vi "Inverter LUT UI - Standalone.vi"() -> ()   [LabVIEW 2019]
doc: "Developed by Kevin Thompson\nkevin@thompsonengineering.net\n\nCopyright 2020\nThompson Engineering, LLC"
uses:
  DataTypes/inverter offset range--cluster.ctl
  DataTypes/inverter gain range--cluster.ctl
  <vilib>/TELLC/Dynamic CVT API/TD Dynamic CVT DVR--ref.ctl
  DataTypes/inverter info v2--cluster.ctl
  DataTypes/Inverter database record v2--cluster.ctl
  DataTypes/Inverter LUT v2--cluster.ctl
panel:
  out "last updated":string="Micro < 500W"
  in  "offset range":T1={"offset max"=3000.0, "offset min"=2000.0, "offset increment"=0.0} caption="Offset Range"
  in  "gain range":T2={"gain max"=4000.0, "gain min"=3000.0, "gain increment"=100.0} caption="Gain Range"
  in  "resistance 3 phase":dbl
  in  "resistance single phase":dbl=50.0
  in  "minimum current":dbl
  in  "power level":dbl
  in  "set flag":u16(ring) items=["False", "True"]
  in  "gain actual":dbl
  in  "offset actual":dbl
  in  "inverter Info":T3
  in  "type":string="Micro < 500W"
  in  "name":string="Inverter-01"
  in  "Inverter List":i32(listbox)
  in  "AddRec":bool
  in  "DeleteRec":bool
  out "CurrRec":i32 caption="Current\nRecord Index"
  out "Total":i32 caption="Total Inverter\nRecords"
  in  "LUT File":path
  in  "Load":bool
  in  "UpdateRec":bool
  in  "Exit":bool
  # "Inverter Record"
  # "auto filled"
  # "INVERTER  DATABASE  EDITOR"
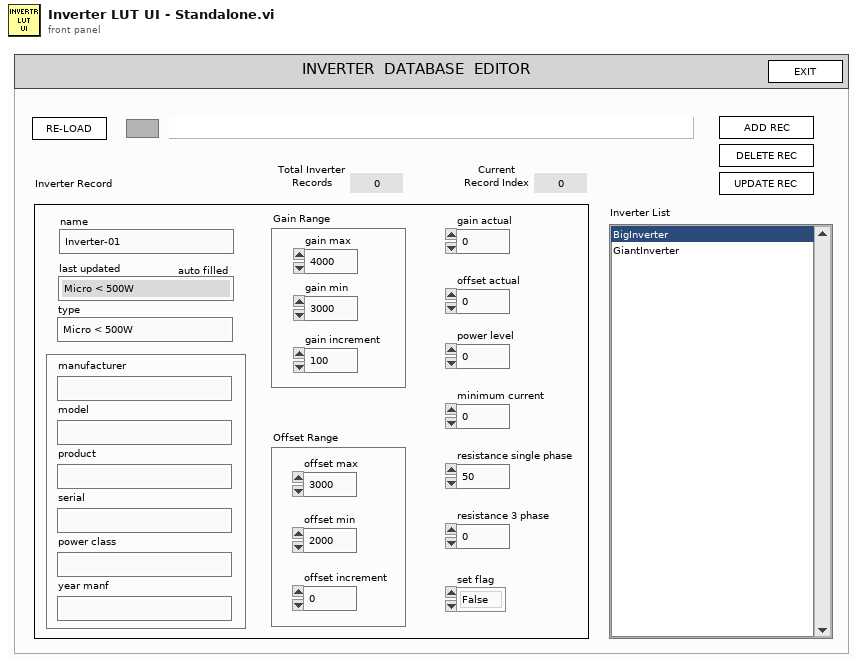
[diagram p1: front panel]
types:
  T1 = typedef "inverter offset range--cluster.ctl" = cluster{"offset max":dbl, "offset min":dbl, "offset increment":dbl}
  T2 = typedef "inverter gain range--cluster.ctl" = cluster{"gain max":dbl, "gain min":dbl, "gain increment":dbl}
  T3 = typedef "inverter info v2--cluster.ctl" = cluster{"manufacturer":string, "model":string, "product":string, "serial":string, "power class":string, "year manf":string}
  T4 = typedef "Inverter LUT v2--cluster.ctl" = cluster{"Inverter Records":T5[]}
  T5 = typedef "Inverter database record v2--cluster.ctl" = cluster{"name":string, "last updated":timestamp, "type":string, "inverter Info":T3, "gain range":T2, "offset range":T1, "gain actual":dbl, "offset actual":dbl, "power level":dbl, "minimum current":dbl, "resistance single phase":dbl, "resistance 3 phase":dbl, "set flag":u16}
  T6 = enum32{"invalid app kind", "Development System", "Run Time System", "Student Edition", "Embedded LabVIEW", "Evaluation", "Custom"}
  T7 = enum32{"Invalid", "Default", "Floating", "Floating/Auto-Hide", "Modal"}
  T8 = enum32{"Invalid", "Standard", "Closed", "Hidden", "Minimized", "Maximized"}
  T9 = typedef "TD Dynamic CVT DVR--ref.ctl" = refnum<data-value>
  T10 = cluster{"Core":cluster{"Current VI Reference":refnum<vi>, "Close Panel on Exit?":bool}, "CurrInverterRec":T5, "All Records":T5[], "InverterLUT Dict":T9}
  T11 = cluster{"Current VI Reference":refnum<vi>, "Close Panel on Exit?":bool}
  T12 = enum16{"Left Button", "Center Button", "Right Button", "Window Close"}
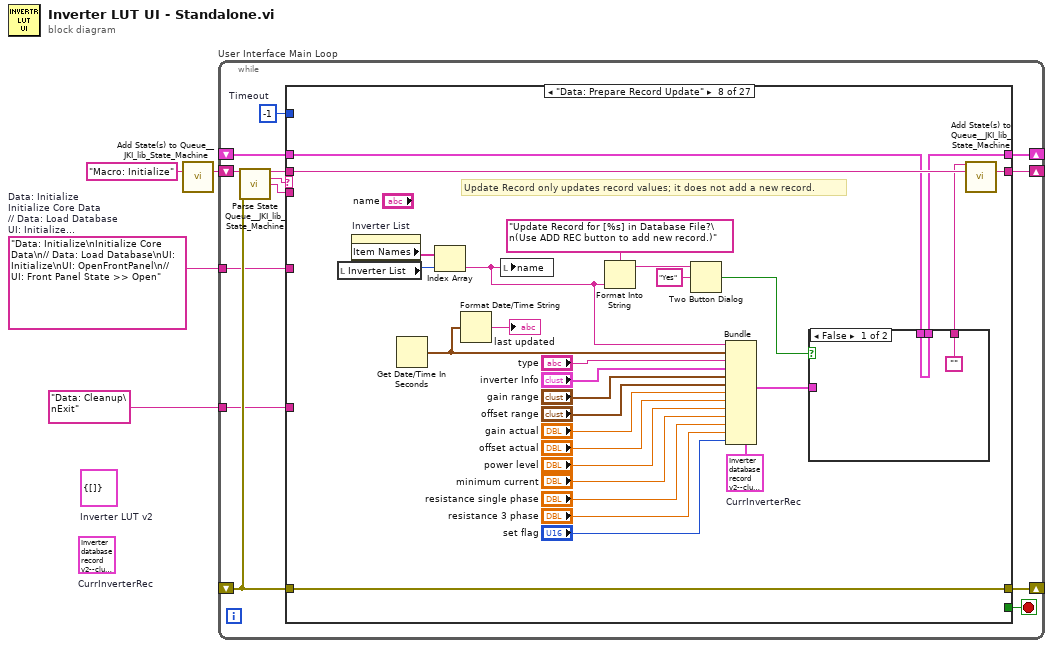
[diagram p0: block diagram]
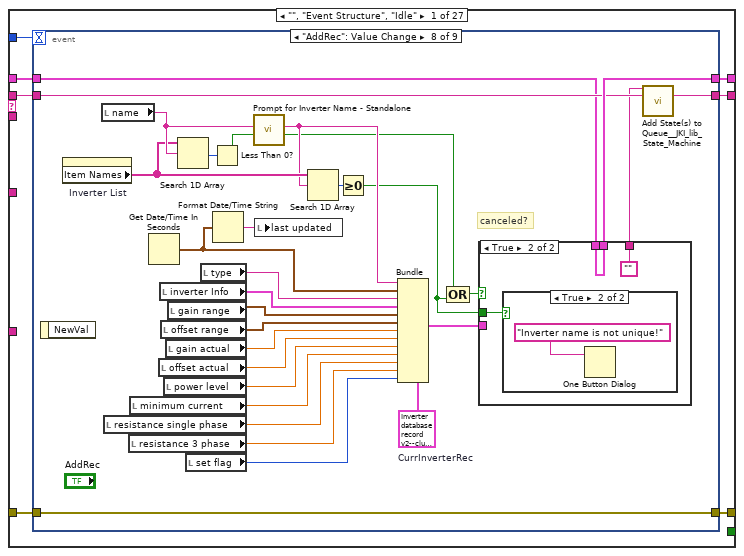
[diagram p2: hidden frame]
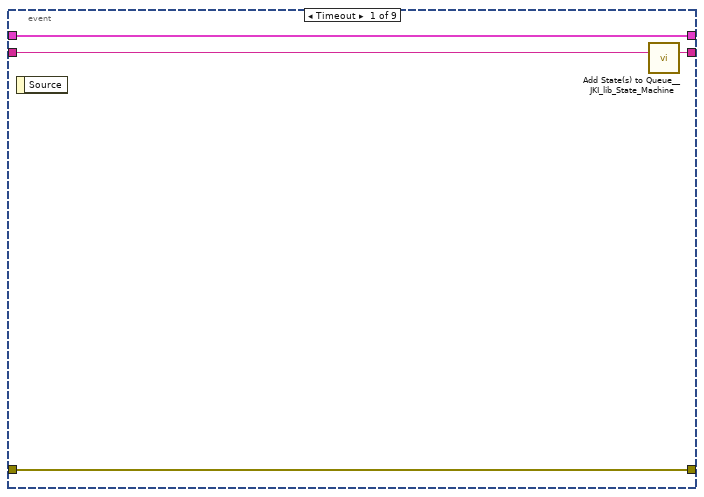
[diagram p3: hidden frame]
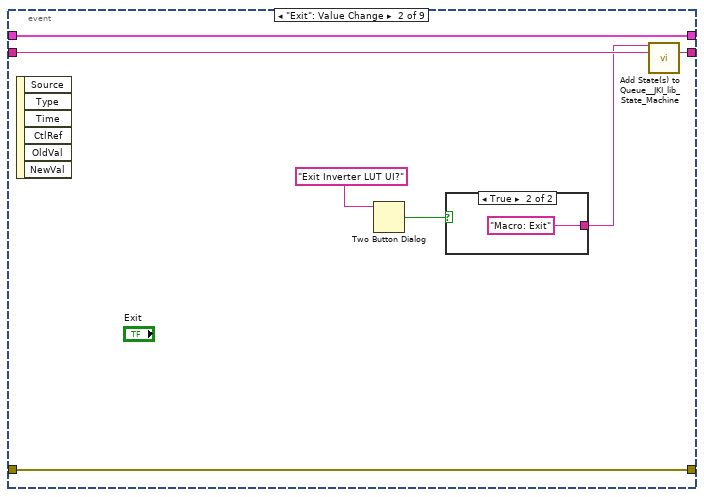
[diagram p4: hidden frame]
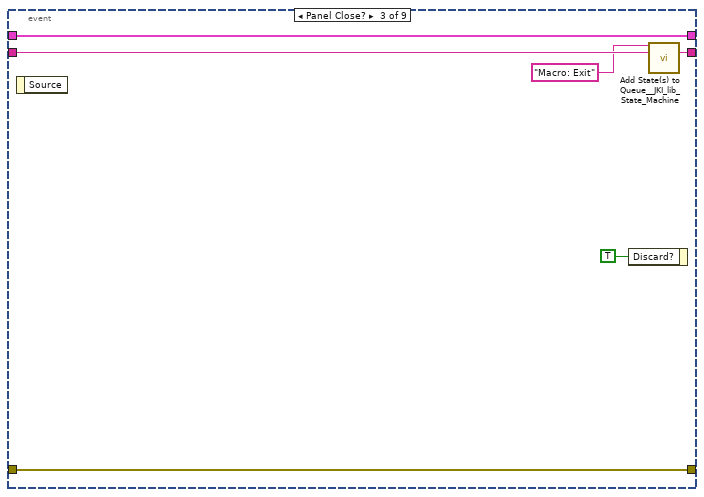
[diagram p6: hidden frame]
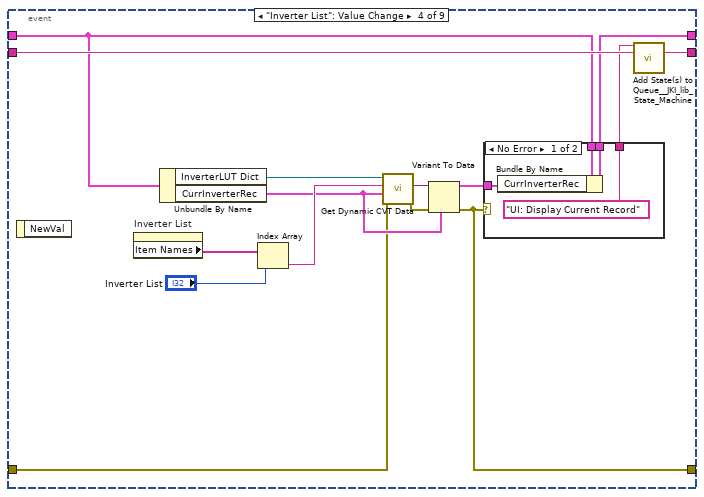
[diagram p7: hidden frame]
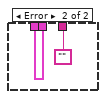
[diagram p8: hidden frame]
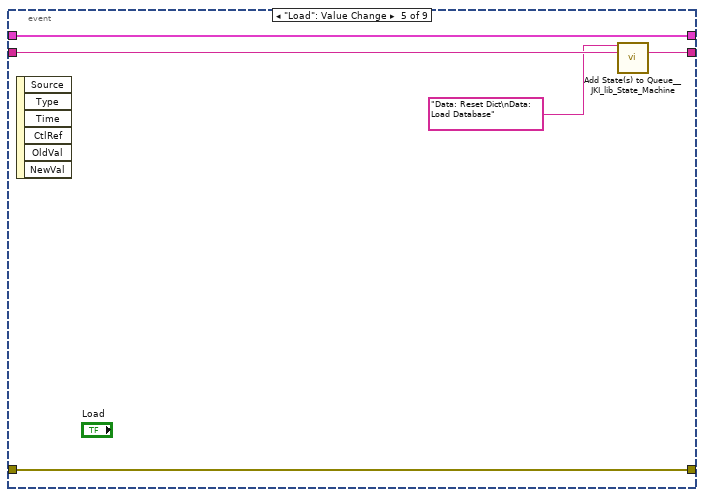
[diagram p9: hidden frame]
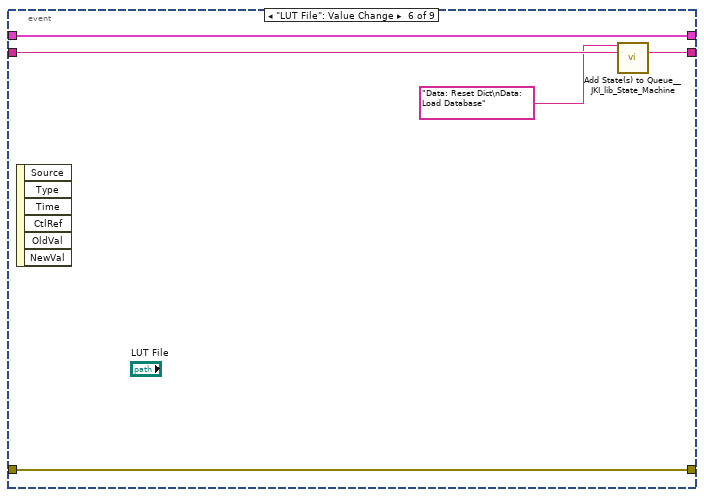
[diagram p10: hidden frame]
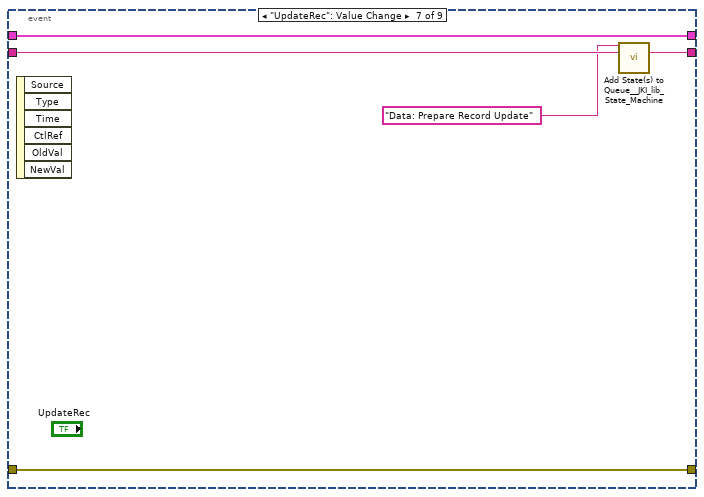
[diagram p11: hidden frame]
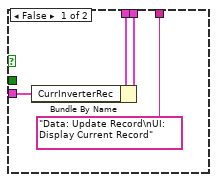
[diagram p12: hidden frame]
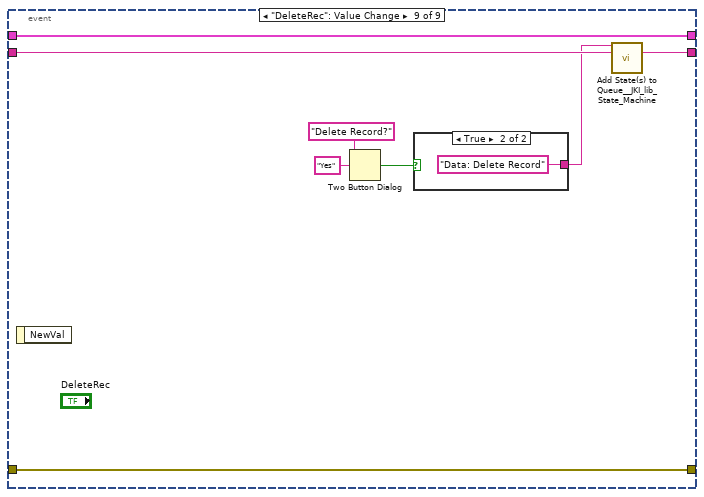
[diagram p14: hidden frame]
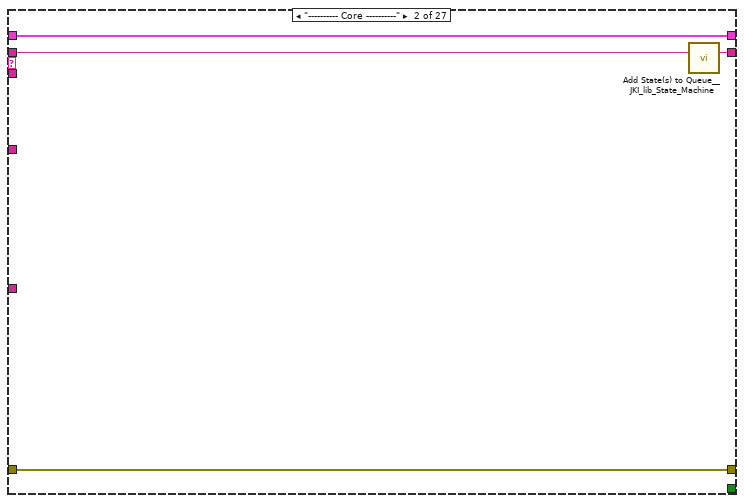
[diagram p16: hidden frame]
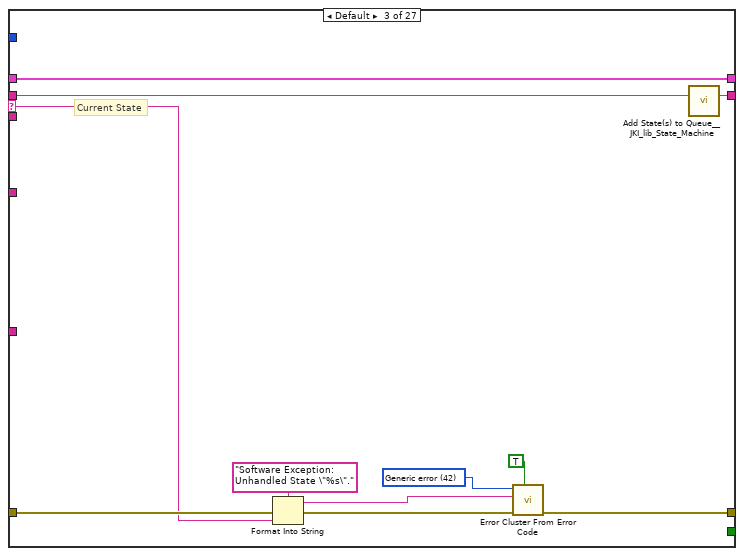
[diagram p17: hidden frame]
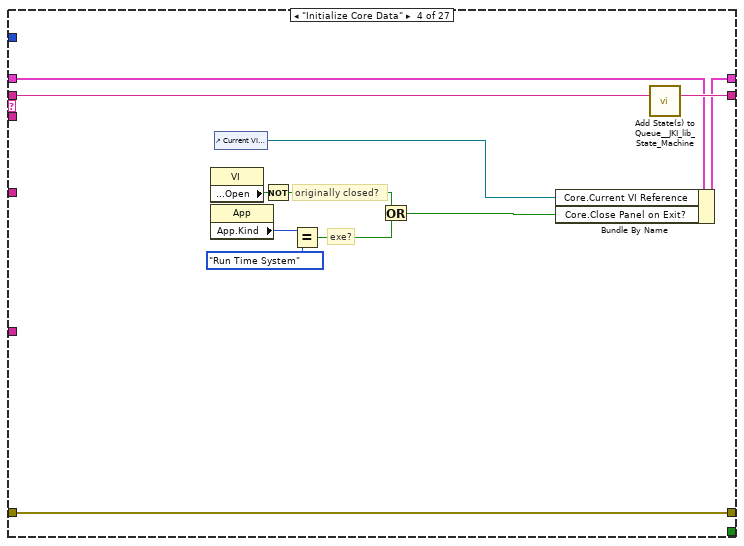
[diagram p18: hidden frame]
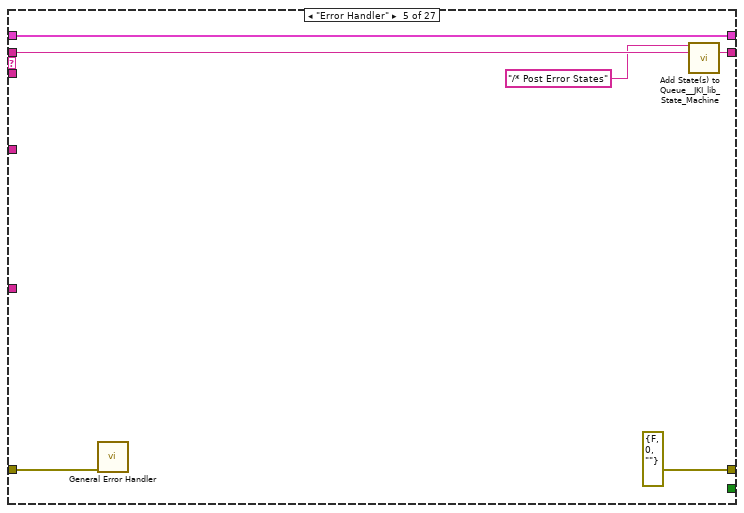
[diagram p19: hidden frame]
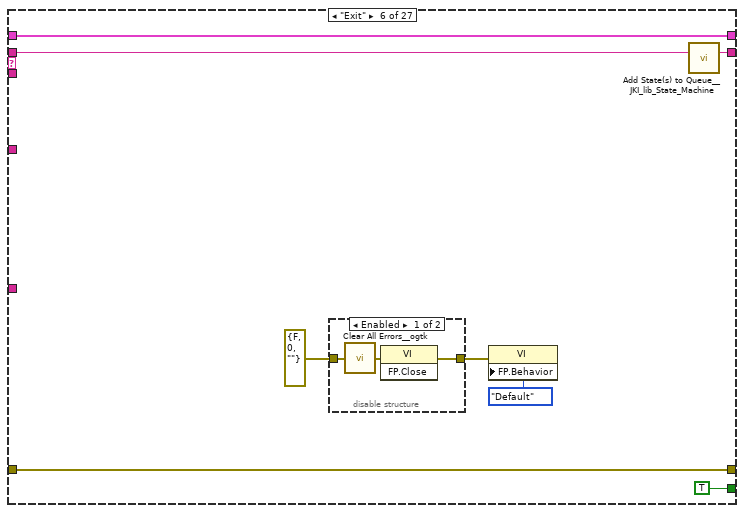
[diagram p20: hidden frame]
diagram:
  (unwired) T4 {"Inverter Records"=[]}  # Inverter LUT v2
  (unwired) T5 {"name"="", "last updated"=timestamp(0 s since 1904-01-01), "type"="", "inverter Info"={"manufacturer"="", "model"="", "product"="", "serial"="", "power class"="", "year manf"=""}, "gain range"={"gain max"=0.0, "gain min"=0.0, "gain increment"=0.0}, "offset range"={"offset max"=0.0, "offset min"=0.0, "offset increment"=0.0}, "gain actual"=0.0, "offset actual"=0.0, "power level"=0.0, "minimum current"=0.0, "resistance single phase"=0.0, "resistance 3 phase"=0.0, "set flag"=0}  # CurrInverterRec
  w2 = "Data: Initialize\nInitialize Core Data\n// Data: Load Database\nUI: Initialize\nUI: OpenFrontPanel\n// UI: Front Panel State >> Open"  # Data: Initialize Initialize Core Data // Data: Load Database UI: Initialize UI: OpenFrontPanel // UI: Front Panel State >> Open
  n1 = call <vilib>:"Add State(s) to Queue__JKI_lib_State_Machine.vi"("State(s) in (\"\")"="Macro: Initialize") -> ("States Out"=w4:string)  [unwired: 14 in]
  n2 = while "User Interface Main Loop" {
    shift-right: [w10] -> _
    shift-left: _ -> [w9]
    shift-right: [w13] -> _
    shift-left: _ -> [w7]
    shift-right: [w12] -> _
    shift-left: w4 -> [w14]
    tunnel: w2 -> [w6]
    tunnel: "Data: Cleanup\nExit" -> [w5]
    stop <- w11 stop-if-true
    w8 = -1  # Timeout
    n3 = call <vilib>:"Parse State Queue__JKI_lib_State_Machine.vi"("State Queue"=w14, "Error In (no error)"=w7) -> ("Remaining States"=w16:string, "Current State"=w17:string, "Arguments"=w15:string)  [unwired: 11 in]
    n4 = case shown="\"Data: Prepare Record Update\"" w17 {
      selector: w17 -> [_ _ w130 _ _ _ _ _ _ _ _ _ _ _ _ _ _ _ _ _ _ _ _ _ _ _ _]
      tunnel: w16 -> [w24 w129 w134 w152 w158 w166 w174 w202 w214 w234 w263 w300 w337 w346 w350 w359 w383 w405 w423 w429 w440 w466 w471 w481 w485 w489 w493]
      tunnel: w15 -> [_ _ _ _ _ _ _ _ _ _ _ _ _ _ _ _ _ _ _ w424 w434 _ _ _ _ _ _]
      tunnel: w9 -> [w22 w126 w132 w143 w155 w164 w171 w196 w212 w223 w261 w292 _ w341 w347 w356 w369 w391 w415 w427 w436 w463 w468 w478 w482 w486 w490]
      tunnel: [w21 w127 w136 w149 errorcluster {"status"=FALSE, "code"=0, "source"=""} ("error out") w163 w172 w200 w210 w218 w249 w279 w334 w342 w348 w357 w381 w403 w412 w425 w437 w464 w469 w479 w483 w487 w491] -> w13
      tunnel: w7 -> [w20 w127 w135 w149 w154 w163 w172 w200 w209 w217 w258 w293 w334 w343 w348 w357 w381 w403 w411 w426 w438 w464 w469 w479 w483 w487 w491]
      tunnel: [w23 w128 w133 w151 w157 w165 w173 w201 w213 w233 w262 w299 w336 w345 w349 w358 w382 w404 w422 w428 w439 w465 w470 w480 w484 w488 w492] -> w12
      tunnel: [_ _ _ _ _ TRUE _ _ _ _ _ _ _ _ _ _ _ _ _ _ _ _ _ _ _ _ _] -> w11
      tunnel: [w19 w126 w132 w150 w155 w164 w171 w195 w212 w224 w261 w295 w335 w341 w347 w356 w369 w391 w415 w427 w436 w463 w468 w478 w482 w486 w490] -> w10
      tunnel: w8 -> [w18 _ _ _ _ _ _ _ _ _ _ _ _ _ _ _ _ _ _ _ _ _ _ _ _ _ _]
      tunnel: w6 -> [_ _ _ _ _ _ _ _ _ _ _ _ _ _ _ _ _ _ _ _ _ _ w467 _ _ _ _]
      tunnel: w5 -> [_ _ _ _ _ _ _ _ _ _ _ _ _ _ _ _ _ _ _ _ _ _ _ w472 _ _ _]
      frame "", "Event Structure", "Idle" {
        n5 = event shown="[7] \"AddRec\": Value Change" {
          selector: _ -> [_ _ _ _ _ _ _ _ _]
          dyn-events: _ -> [_ _ _ _ _ _ _ _ _]
          timeout: w18 -> [_ _ _ _ _ _ _ _ _]
          tunnel: w24 -> [w28 w35 w42 w50 w65 w71 w76 w104 w119]
          tunnel: [w27 w34 w41 w51 w66 w72 w77 w105 w120] -> w23
          tunnel: w22 -> [w25 w32 w39 w47 w67 w69 w75 w88 w123]
          tunnel: [w26 w33 w40 w45 w68 w73 w78 w108 w124] -> w21
          tunnel: w20 -> [w26 w33 w40 w44 w68 w73 w78 w108 w124]
          tunnel: [w25 w32 w39 w48 w67 w69 w75 w107 w123] -> w19
          event Timeout {
            n6 = event-data() -> ()  [unwired: 1 in, 1 out]
            n7 = call <vilib>:"Add State(s) to Queue__JKI_lib_State_Machine.vi"("State(s) in (\"\")"=w28) -> ("States Out"=w27:string)  [unwired: 14 in]
          }
          event "Exit": Value Change {
            n8 = event-data() -> ()  [unwired: 1 in, 6 out]
            n9 = Two Button Dialog(message="Exit Inverter LUT UI?") -> (T button?=w29:bool)  [unwired: 2 in]
            n10 = case shown="True" w29 {
              tunnel: [_ "Macro: Exit"] -> w31
              frame False {
              }
              frame True {
              }
            }
            n11 = call <vilib>:"Add State(s) to Queue__JKI_lib_State_Machine.vi"("State(s) in Front (\"\")"=w31, "State(s) in (\"\")"=w35) -> ("States Out"=w34:string)  [unwired: 13 in]
          }
          event Panel Close? {
            n12 = event-data() -> ()  [unwired: 1 in, 1 out]
            n13 = event-data("Discard?"=TRUE) -> ()  [unwired: 1 in, 1 out]
            n14 = call <vilib>:"Add State(s) to Queue__JKI_lib_State_Machine.vi"("State(s) in Front (\"\")"="Macro: Exit", "State(s) in (\"\")"=w42) -> ("States Out"=w41:string)  [unwired: 13 in]
          }
          event "Inverter List": Value Change {
            n15 = event-data() -> ()  [unwired: 1 in, 1 out]
            n16 = property on="Inverter List" class="LstBox (strict)"() -> ("Item Names"=w57:string[])  [unwired: 2 in, 2 out]
            n17 = Unbundle By Name(w47) -> ("InverterLUT Dict"=w56:T9, "CurrInverterRec"=w53:T5)
            n18 = Index Array(array=w57, index="Inverter List") -> (element=w55:string)
            n19 = call <vilib>:"Get Dynamic CVT Data.vi"("error in (no error)"=w44, "default value (empty variant)"=w53, "DataName"=w55, "dCVT DVR"=w56) -> ("error out"=w54:errorcluster, "value"=w52:variant)  [unwired: 4 in, 2 out]
            n20 = Variant To Data(error in=w54, type=w53, Variant=w52) -> (data=w49:T5, error out=w45:errorcluster)
            n21 = case shown="No Error" w45 {
              tunnel: w49 -> [w61 _]
              tunnel: [w60 w63] -> w48
              tunnel: w47 -> [w59 w63]
              tunnel: ["UI: Display Current Record" ""] -> w46
              frame No Error {
                n22 = Bundle By Name(cluster=w59, "CurrInverterRec"=w61) -> (w60:T10)
              }
              frame Error {
              }
            }
            n23 = call <vilib>:"Add State(s) to Queue__JKI_lib_State_Machine.vi"("State(s) in Front (\"\")"=w46, "State(s) in (\"\")"=w50) -> ("States Out"=w51:string)  [unwired: 13 in]
          }
          event "Load": Value Change {
            n24 = event-data() -> ()  [unwired: 1 in, 6 out]
            n25 = call <vilib>:"Add State(s) to Queue__JKI_lib_State_Machine.vi"("State(s) in Front (\"\")"="Data: Reset Dict\nData: Load Database", "State(s) in (\"\")"=w65) -> ("States Out"=w66:string)  [unwired: 13 in]
          }
          event "LUT File": Value Change {
            n26 = event-data() -> ()  [unwired: 1 in, 6 out]
            n27 = call <vilib>:"Add State(s) to Queue__JKI_lib_State_Machine.vi"("State(s) in Front (\"\")"="Data: Reset Dict\nData: Load Database", "State(s) in (\"\")"=w71) -> ("States Out"=w72:string)  [unwired: 13 in]
          }
          event "UpdateRec": Value Change {
            n28 = event-data() -> ()  [unwired: 1 in, 6 out]
            n29 = call <vilib>:"Add State(s) to Queue__JKI_lib_State_Machine.vi"("State(s) in Front (\"\")"="Data: Prepare Record Update", "State(s) in (\"\")"=w76) -> ("States Out"=w77:string)  [unwired: 13 in]
          }
          event "AddRec": Value Change {
            w102 = T5 {"name"="", "last updated"=timestamp(0 s since 1904-01-01), "type"="", "inverter Info"={"manufacturer"="", "model"="", "product"="", "serial"="", "power class"="", "year manf"=""}, "gain range"={"gain max"=0.0, "gain min"=0.0, "gain increment"=0.0}, "offset range"={"offset max"=0.0, "offset min"=0.0, "offset increment"=0.0}, "gain actual"=0.0, "offset actual"=0.0, "power level"=0.0, "minimum current"=0.0, "resistance single phase"=0.0, "resistance 3 phase"=0.0, "set flag"=0}  # CurrInverterRec
            # "canceled?"
            n30 = event-data() -> ()  [unwired: 1 in, 1 out]
            n31 = property on="Inverter List" class="LstBox (strict)"() -> ("Item Names"=w84:string[])  [unwired: 2 in, 2 out]
            n32 = local read "name"() -> (w87:string)
            n33 = local read "resistance single phase"() -> (w99:dbl)
            n34 = local read "resistance 3 phase"() -> (w100:dbl)
            n35 = local read "minimum current"() -> (w98:dbl)
            n36 = Get Date/Time In Seconds() -> (seconds since 1Jan1904=w90:timestamp)
            n37 = local read "offset actual"() -> (w96:dbl)
            n38 = local read "inverter Info"() -> (w92:T3)
            n39 = local read "offset range"() -> (w94:T1)
            n40 = local read "power level"() -> (w97:dbl)
            n41 = local read "gain actual"() -> (w95:dbl)
            n42 = local read "gain range"() -> (w93:T2)
            n43 = Search 1D Array(1D array=w84, element=w87) -> (index of element=w86:i32)  [unwired: 1 in]
            n44 = local read "set flag"() -> (w101:u16)
            n45 = local read "type"() -> (w91:string)
            n46 = Less Than 0?(x=w86) -> (x < 0?=w85:bool)
            n47 = Format Date/Time String(seconds (now)=w90) -> (date/time string=w89:string)  [unwired: 2 in]
            n48 = call "Prompt for Inverter Name - Standalone.vi"("bypass (F)"=w85, "Name"=w87) -> ("canceled"=w80:bool, "name out"=w83:string)  [unwired: 7 in, 1 out]
            n49 = local write "last updated"(w89) -> ()
            n50 = Search 1D Array(1D array=w84, element=w83) -> (index of element=w82:i32)  [unwired: 1 in]
            n51 = Greater Or Equal To 0?(x=w82) -> (x >= 0?=w79:bool)
            n52 = Bundle(cluster=w102, "name"=w83, "last updated"=w90, "type"=w91, "inverter Info"=w92, "gain range"=w93, "offset range"=w94, "gain actual"=w95, "offset actual"=w96, "power level"=w97, "minimum current"=w98, "resistance single phase"=w99, "resistance 3 phase"=w100, "set flag"=w101) -> (w106:T5)
            n53 = Compound Arithmetic op=OR(w80, w79) -> (w81:bool)
            n54 = case shown="True" w81 {
              tunnel: [w112 w115] -> w107
              tunnel: w88 -> [w111 w115]
              tunnel: w106 -> [w110 _]
              tunnel: ["Data: Update Record\nUI: Display Current Record" ""] -> w103
              tunnel: w79 -> [_ w113]
              frame False {
                n55 = Bundle By Name(cluster=w111, "CurrInverterRec"=w110) -> (w112:T10)
              }
              frame True {
                n56 = case shown="True" w113 {
                  frame False {
                  }
                  frame True {
                    n57 = One Button Dialog(message="Inverter name is not unique!") -> ()  [unwired: 1 in, 1 out]
                  }
                }
              }
            }
            n58 = call <vilib>:"Add State(s) to Queue__JKI_lib_State_Machine.vi"("State(s) in Front (\"\")"=w103, "State(s) in (\"\")"=w104) -> ("States Out"=w105:string)  [unwired: 13 in]
          }
          event "DeleteRec": Value Change {
            n59 = event-data() -> ()  [unwired: 1 in, 1 out]
            n60 = Two Button Dialog(message="Delete Record?", 2:"Yes" ("T button name (\"OK\")")) -> (T button?=w117:bool)  [unwired: 1 in]
            n61 = case shown="True" w117 {
              tunnel: [_ "Data: Delete Record"] -> w118
              frame False {
              }
              frame True {
              }
            }
            n62 = call <vilib>:"Add State(s) to Queue__JKI_lib_State_Machine.vi"("State(s) in Front (\"\")"=w118, "State(s) in (\"\")"=w119) -> ("States Out"=w120:string)  [unwired: 13 in]
          }
        }
      }
      frame "---------- Core ----------" {
        n63 = call <vilib>:"Add State(s) to Queue__JKI_lib_State_Machine.vi"("State(s) in (\"\")"=w129) -> ("States Out"=w128:string)  [unwired: 14 in]
      }
      frame Default {
        w139 = 42 items=["No error", "Argument error", "Memory is full", "Out of zone", "End of file", "File already open", "Generic file I/O error", "File not found", "File permission error", "Disk is full", "Duplicate path", "Too many files open", "System feature not enabled", "Resource file not found", "Cannot add resource", "Resource not found", "Image not found", "Image memory error", "Pen does not exist", "Config type invalid", "Config token not found", "Config parse error", "Config memory error", "Bad external code format", "Bad external code offset", "External code not present", "Null window", "Destroy window error", "Null menu", "Print aborted", "Bad print record", "Print driver error", "Windows error during printing", "Memory error during printing", "Print dialog error", "Generic print error", "Invalid device refnum", "Device not found", "Device parameter error", "Device unit error", "Cannot open device", "Device call aborted", "Generic error", "Cancelled by user", "Object ID too low", "Object ID too high", "Object not in heap", "Unknown heap", "Unknown object (invalid DefProc)", "Unknown object (DefProc not in table)", "Message out of range", "Invalid (null) method", "Unknown message", "Manager call not supported", "Bad address", "Network operation in progress", "Network operation timed out", "Connection is busy", "Network attribute not supported", "Network error", "Address in use", "System out of memory", "Connection aborted", "Connection refused", "Not connected", "Already connected", "Connection closed", "Initialization error (interapplication manager)", "Bad occurrence", "Wait on unbound occurrence handler", "Occurrence queue overflow", "Datalog type conflict", "Unused", "Unrecognized type (interapplication manager)", "Memory corrupt", "Failed to make temporary DLL", "Old CIN version", "Drag socket not found", "Failed to load drop-object", "Failed to register OLE object", "Failed to release OLE object", "Format specifier type mismatch", "Unknown format specifier", "Too few format specifiers", "Too many format specifiers", "Scan failed", "Newer CIN version", "Error converting to variant", "Runtime menu error", "Password tampered", "Variant attribute not found", "Incompatible variant data type", "Event data is not available", "Event Store is not present", "Occurrence is not found", "Event Queue is not created", "Event info is not available", "Refnum passed is NULL", "Error retrieving Class GUID", "Error retrieving CoClass GUID", "Error retrieving TypeLib GUID.", "Bad built application magic bytes.", "Specific driver is different from the specific driver associated with the Logical Name.", "There is no session opened to the class driver.", "Max Error", "MAX - Error with config objects", "MAX - Error loading configuration", "MAX - Group not supported"]
        # "Current State"
        n64 = Format Into String(format string="Software Exception: Unhandled State \"%s\"." ("message"), error in=w135, w130) -> (resulting string=w138:string, error out=w137:errorcluster)  [unwired: 1 in]
        n65 = call <vilib>:"Error Cluster From Error Code.vi"("show call chain? (False)"=TRUE, "error in (no error)"=w137, "error message (\"\")"=w138, "error code (0)"=w139) -> ("error out"=w136:errorcluster)  [unwired: 5 in]
        n66 = call <vilib>:"Add State(s) to Queue__JKI_lib_State_Machine.vi"("State(s) in (\"\")"=w134) -> ("States Out"=w133:string)  [unwired: 14 in]
      }
      frame "Initialize Core Data" {
        # "originally closed?"
        # "exe?"
        n67 = property class="VI"() -> ("Front Panel.Open"=w148:bool)  [unwired: 2 in, 2 out]
        n68 = property class="App"() -> ("App.Kind"=w147:T6)  [unwired: 2 in, 2 out]
        n69 = control-ref of="Current VI Reference"() -> (w141:refnum<vi>)
        n70 = Not(x=w148) -> (.not. x?=w145:bool)
        n71 = Equal?(x=w147, y=T6."Run Time System" ("Application:Kind")) -> (x = y?=w144:bool)
        n72 = Or(x=w145, y=w144) -> (x .or. y?=w142:bool)
        n73 = Bundle By Name(cluster=w143, "Core.Current VI Reference"=w141, "Core.Close Panel on Exit?"=w142) -> (w150:T10)
        n74 = call <vilib>:"Add State(s) to Queue__JKI_lib_State_Machine.vi"("State(s) in (\"\")"=w152) -> ("States Out"=w151:string)  [unwired: 14 in]
      }
      frame "Error Handler" {
        n75 = call <vilib>:"General Error Handler.vi"("error in (no error)"=w154) -> ()  [unwired: 10 in, 5 out]
        n76 = call <vilib>:"Add State(s) to Queue__JKI_lib_State_Machine.vi"("State(s) in Front (\"\")"="/* Post Error States", "State(s) in (\"\")"=w158) -> ("States Out"=w157:string)  [unwired: 13 in]
      }
      frame "Exit" {
        n77 = disable-structure shown="Enabled" {
          disable-tunnel: [w169 w170] -> w161
          disable-tunnel: errorcluster {"status"=FALSE, "code"=0, "source"=""} ("Error In") -> [w167 w170]
          frame Enabled {
            n78 = call <userlib>:"Clear All Errors__ogtk.vi"("Error In"=w167) -> ("Error Out"=w168:errorcluster)  [unwired: 3 in]
            n79 = invoke class="VI" method="FP.Close"(error in=w168) -> (error out=w169:errorcluster)  [unwired: 2 in, 2 out]
          }
          frame Disabled {
          }
        }
        n80 = property class="VI"(error in=w161, "FP.Behavior"=T7."Default" ("Front Panel Window:Behavior")) -> ()  [unwired: 1 in, 2 out]
        n81 = call <vilib>:"Add State(s) to Queue__JKI_lib_State_Machine.vi"("State(s) in (\"\")"=w166) -> ("States Out"=w165:string)  [unwired: 14 in]
      }
      frame "---------- Data ----------" {
        n82 = call <vilib>:"Add State(s) to Queue__JKI_lib_State_Machine.vi"("State(s) in (\"\")"=w174) -> ("States Out"=w173:string)  [unwired: 14 in]
      }
      frame "Data: Prepare Record Update" {
        w189 = T5 {"name"="", "last updated"=timestamp(0 s since 1904-01-01), "type"="", "inverter Info"={"manufacturer"="", "model"="", "product"="", "serial"="", "power class"="", "year manf"=""}, "gain range"={"gain max"=0.0, "gain min"=0.0, "gain increment"=0.0}, "offset range"={"offset max"=0.0, "offset min"=0.0, "offset increment"=0.0}, "gain actual"=0.0, "offset actual"=0.0, "power level"=0.0, "minimum current"=0.0, "resistance single phase"=0.0, "resistance 3 phase"=0.0, "set flag"=0}  # CurrInverterRec
        # "Update Record only updates record values; it does not add a new record."
        n83 = local read "Inverter List"() -> (w193:i32)
        n84 = property on="Inverter List" class="LstBox (strict)"() -> ("Item Names"=w192:string[])  [unwired: 2 in, 2 out]
        n85 = Get Date/Time In Seconds() -> (seconds since 1Jan1904=w175:timestamp)
        n86 = Index Array(array=w192, index=w193) -> (element=w177:string)
        n87 = Format Date/Time String(seconds (now)=w175) -> (date/time string=→"last updated":string)  [unwired: 2 in]
        n88 = local write "name"(w177) -> ()
        n89 = Format Into String(format string="Update Record for [%s] in Database File?\n(Use ADD REC button to add new record.)" ("message"), w177) -> (resulting string=w190:string)  [unwired: 2 in, 1 out]
        n90 = Two Button Dialog(message=w190, 2:"Yes" ("T button name (\"OK\")")) -> (T button?=w198:bool)  [unwired: 1 in]
        n91 = Bundle(cluster=w189, "name"=w177, "last updated"=w175, "type"="type", "inverter Info"="inverter Info", "gain range"="gain range", "offset range"="offset range", "gain actual"="gain actual", "offset actual"="offset actual", "power level"="power level", "minimum current"="minimum current", "resistance single phase"="resistance single phase", "resistance 3 phase"="resistance 3 phase", "set flag"="set flag") -> (w199:T5)
        n92 = case shown="False" w198 {
          tunnel: [w204 w208] -> w195
          tunnel: w196 -> [w204 w207]
          tunnel: w199 -> [_ w206]
          tunnel: ["" "Data: Update Record"] -> w194
          frame False {
          }
          frame True {
            n93 = Bundle By Name(cluster=w207, "CurrInverterRec"=w206) -> (w208:T10)
          }
        }
        n94 = call <vilib>:"Add State(s) to Queue__JKI_lib_State_Machine.vi"("State(s) in Front (\"\")"=w194, "State(s) in (\"\")"=w202) -> ("States Out"=w201:string)  [unwired: 13 in]
      }
      frame "Data: Reset Dict" {
        n95 = Unbundle By Name(w212) -> ("InverterLUT Dict"=w211:T9)
        n96 = call <vilib>:"Delete ALL Dynamic CVT Data.vi"("error in (no error)"=w209, "dCVT DVR"=w211) -> ("error out"=w210:errorcluster)  [unwired: 8 in, 1 out]
        n97 = call <vilib>:"Add State(s) to Queue__JKI_lib_State_Machine.vi"("State(s) in (\"\")"=w214) -> ("States Out"=w213:string)  [unwired: 14 in]
      }
      frame "Data: Delete Record" {
        w215 = T5 {"name"="", "last updated"=timestamp(0 s since 1904-01-01), "type"="", "inverter Info"={"manufacturer"="", "model"="", "product"="", "serial"="", "power class"="", "year manf"=""}, "gain range"={"gain max"=0.0, "gain min"=0.0, "gain increment"=0.0}, "offset range"={"offset max"=0.0, "offset min"=0.0, "offset increment"=0.0}, "gain actual"=0.0, "offset actual"=0.0, "power level"=0.0, "minimum current"=0.0, "resistance single phase"=0.0, "resistance 3 phase"=0.0, "set flag"=0}  # CurrInverterRec
        n98 = Unbundle By Name(w223) -> ("InverterLUT Dict"=w232:T9, "CurrInverterRec"=w230:T5)
        n99 = Unbundle By Name(w230) -> ("name"=w231:string)
        n100 = call <vilib>:"Delete Dynamic CVT Data.vi"("error in (no error)"=w217, "DataName"=w231, "dCVT DVR"=w232) -> ("error out"=w228:errorcluster, "CVT DVR out"=w229:T9)  [unwired: 6 in, 1 out]
        n101 = call <vilib>:"Get ALL Dynamic CVT Data.vi"("error in (no error)"=w228, "dCVT DVR"=w229) -> ("error out"=w220:errorcluster, "NameArray"=w225:string[], "ValueArray"=w227:variant[])  [unwired: 6 in, 1 out]
        n102 = Index Array(array=w227) -> (element=w226:variant)  [unwired: 1 in]
        n103 = property on="Inverter List" class="LstBox (strict)"(error in=w220, "Item Names"=w225) -> (error out=w221:errorcluster)  [unwired: 1 in, 1 out]
        n104 = Variant To Data(error in=w220, type=w215, Variant=w226) -> (data=w222:T5, error out=w219:errorcluster)
        n105 = Bundle By Name(cluster=w223, "CurrInverterRec"=w222) -> (w224:T10)
        n106 = flat-sequence {
          tunnel: w221 -> [w237]
          tunnel: w219 -> [w236]
          tunnel: [w235] -> w218
          frame #0 {
            n107 = Merge Errors(w236, w237) -> (w235:errorcluster)
            n108 = local write "Inverter List"(0 ("Inverter List")) -> ()
          }
        }
        n109 = call <vilib>:"Add State(s) to Queue__JKI_lib_State_Machine.vi"("State(s) in Front (\"\")"="Data: Update Record\nUI: Display Current Record", "State(s) in (\"\")"=w234) -> ("States Out"=w233:string)  [unwired: 13 in]
      }
      frame "Data: Update Record" {
        w239 = T4 {"Inverter Records"=[]}  # Inverter LUT v2
        n110 = Unbundle By Name(w261) -> ("InverterLUT Dict"=w260:T9, "CurrInverterRec"=w259:T5)
        n111 = Unbundle By Name(w259) -> ("name"=w247:string)
        n112 = call <vilib>:"Set Dynamic CVT Data.vi"("error in (no error)"=w258, "value"=w259, "DataName"=w247, "dCVT DVR"=w260) -> ("error out"=w256:errorcluster, "dCVT DVR out"=w257:T9)  [unwired: 5 in, 1 out]
        n113 = call <userlib>:"Clear All Errors__ogtk.vi"("Error In"=w256) -> ("Error Out"=w241:errorcluster)  [unwired: 3 in]
        n114 = call <vilib>:"Get ALL Dynamic CVT Data.vi"("error in (no error)"=w241, "dCVT DVR"=w257) -> ("error out"=w250:errorcluster, "NameArray"=w248:string[], "ValueArray"=w255:variant[])  [unwired: 6 in, 1 out]
        n115 = call <userlib>:"Clear All Errors__ogtk.vi"("Error In"=w250) -> ("Error Out"=w240:errorcluster)  [unwired: 3 in]
        n116 = for {
          tunnel: w255 -> [w272] mode=indexing
          tunnel: [w271] -> w254 mode=indexing
          n117 = Variant To Data(type=T5 {"name"="", "last updated"=timestamp(0 s since 1904-01-01), "type"="", "inverter Info"={"manufacturer"="", "model"="", "product"="", "serial"="", "power class"="", "year manf"=""}, "gain range"={"gain max"=0.0, "gain min"=0.0, "gain increment"=0.0}, "offset range"={"offset max"=0.0, "offset min"=0.0, "offset increment"=0.0}, "gain actual"=0.0, "offset actual"=0.0, "power level"=0.0, "minimum current"=0.0, "resistance single phase"=0.0, "resistance 3 phase"=0.0, "set flag"=0} ("CurrInverterRec"), Variant=w272) -> (data=w271:T5)  [unwired: 1 in, 1 out]
        }
        n118 = Array Size(array=w248) -> (size(s)=→"Total":i32)
        n119 = Search 1D Array(1D array=w248, element=w247) -> (index of element=w246:i32)  [unwired: 1 in]
        n120 = property on="Inverter List" class="LstBox (strict)"("Item Names"=w248) -> ()  [unwired: 2 in, 2 out]
        n121 = local write "Inverter List"(w246) -> ()
        n122 = Variant To Data(type=T5[] [] ("Inverter Records"), Variant=w254) -> (data=w252:T5[])  [unwired: 1 in, 1 out]
        n123 = Bundle(cluster=w239, "Inverter Records"=w252) -> (w251:T4)
        n124 = local read "LUT File"() -> (w243:path)
        n125 = Empty String/Path?(string/path=w243) -> (empty?=w242:bool)
        n126 = Increment(x=w246) -> (x+1=→"CurrRec":i32)
        n127 = case shown="False" w242 {
          tunnel: w251 -> [w268 _]
          tunnel: w240 -> [w266 w269]
          tunnel: [w265 w269] -> w249
          tunnel: w243 -> [w264 _]
          frame False {
            n128 = call <vilib>:"Easy Write XML File__JKI EasyXML.vi"("error in (no error)"=w266, "Overwrite File? (false)"=TRUE, "LabVIEW Data"=w268, "XML File Path"=w264) -> ("error out"=w265:errorcluster)  [unwired: 6 in, 1 out]
          }
          frame True {
          }
        }
        n129 = call <vilib>:"Add State(s) to Queue__JKI_lib_State_Machine.vi"("State(s) in (\"\")"=w263) -> ("States Out"=w262:string)  [unwired: 14 in]
      }
      frame "Data: Load Database" {
        w284 = T4 {"Inverter Records"=[]}  # Inverter LUT v2
        # "Size difference indicates database file\nhad some duplicate inverter names;\nwhich is not allowed."
        n130 = local read "LUT File"() -> (w285:path)
        n131 = Unbundle By Name(w292) -> ("InverterLUT Dict"=w291:T9)
        n132 = call <vilib>:"Easy Read XML File__JKI EasyXML.vi"("error in (no error)"=w293, "LabVIEW Data (Type)"=w284, "XML File Path"=w285) -> ("error out"=w298:errorcluster, "LabVIEW Data"=w297:variant)  [unwired: 6 in, 1 out]
        n133 = Variant To Data(error in=w298, type=w284, Variant=w297) -> (data=w296:T4, error out=w290:errorcluster)
        n134 = Unbundle(w296) -> ("Inverter Records"=w276:T5[])
        n135 = Array Size(array=w276) -> (size(s)=w275:i32)
        n136 = for {
          tunnel: w276 -> [w316] mode=indexing
          shift-right: [w317] -> w282
          shift-left: w290 -> [w318]
          shift-right: [w319] -> w283
          shift-left: w291 -> [w320]
          n137 = Unbundle By Name(w316) -> ("name"=w315:string)
          n138 = call <vilib>:"Set Dynamic CVT Data.vi"("error in (no error)"=w318, "value"=w316, "DataName"=w315, "dCVT DVR"=w320) -> ("error out"=w317:errorcluster, "dCVT DVR out"=w319:T9)  [unwired: 5 in, 1 out]
        }
        n139 = call <vilib>:"Get ALL Dynamic CVT Data.vi"("error in (no error)"=w282, "dCVT DVR"=w283) -> ("error out"=w280:errorcluster, "NameArray"=w278:string[], "ValueArray"=w281:variant[])  [unwired: 6 in, 1 out]
        n140 = for {
          tunnel: w281 -> [w305] mode=indexing
          tunnel: [w303] -> w277 mode=indexing
          shift-right: [w301] -> w279
          shift-left: w280 -> [w302]
          w304 = T5 {"name"="", "last updated"=timestamp(0 s since 1904-01-01), "type"="", "inverter Info"={"manufacturer"="", "model"="", "product"="", "serial"="", "power class"="", "year manf"=""}, "gain range"={"gain max"=0.0, "gain min"=0.0, "gain increment"=0.0}, "offset range"={"offset max"=0.0, "offset min"=0.0, "offset increment"=0.0}, "gain actual"=0.0, "offset actual"=0.0, "power level"=0.0, "minimum current"=0.0, "resistance single phase"=0.0, "resistance 3 phase"=0.0, "set flag"=0}  # CurrInverterRec
          n141 = Variant To Data(error in=w302, type=w304, Variant=w305) -> (data=w303:T5, error out=w301:errorcluster)
        }
        n142 = Array Size(array=w277) -> (size(s)=w274:i32)
        n143 = local write "Total"(w274) -> ()
        n144 = Not Equal?(x=w275, y=w274) -> (x != y?=w273:bool)
        n145 = Greater Than 0?(x=w274) -> (x > 0?=w289:bool)
        n146 = case shown="True" w289 {
          tunnel: ["" w312] -> w287
          tunnel: [0 ("CurrRec") 1 ("CurrRec")] -> w288
          tunnel: [-1 ("Inverter List") 0 ("Inverter List")] -> w286
          tunnel: w273 -> [_ w309]
          frame False {
          }
          frame True {
            n147 = case shown="True" w309 {
              tunnel: ["UI: Display Current Record" "UI: Warn Dup Records Eliminated"] -> w312
              frame False {
              }
              frame True {
              }
            }
          }
        }
        n148 = Index Array(array=w277) -> (element=w294:T5)  [unwired: 1 in]
        n149 = property on="Inverter List" class="LstBox (strict)"("Item Names"=w278) -> ()  [unwired: 2 in, 2 out]
        n150 = Bundle By Name(cluster=w292, "All Records"=w277, "CurrInverterRec"=w294) -> (w295:T10)
        n151 = local write "CurrRec"(w288) -> ()
        n152 = local write "Inverter List"(w286) -> ()
        n153 = call <vilib>:"Add State(s) to Queue__JKI_lib_State_Machine.vi"("State(s) in Front (\"\")"=w287, "State(s) in (\"\")"=w300) -> ("States Out"=w299:string)  [unwired: 13 in]
      }
      frame "Data: Initialize" {
        w323 = T5 {"name"="", "last updated"=timestamp(0 s since 1904-01-01), "type"="", "inverter Info"={"manufacturer"="", "model"="", "product"="", "serial"="", "power class"="", "year manf"=""}, "gain range"={"gain max"=0.0, "gain min"=0.0, "gain increment"=0.0}, "offset range"={"offset max"=0.0, "offset min"=0.0, "offset increment"=0.0}, "gain actual"=0.0, "offset actual"=0.0, "power level"=0.0, "minimum current"=0.0, "resistance single phase"=0.0, "resistance 3 phase"=0.0, "set flag"=0}  # CurrInverterRec
        w325 = string[] []  # InverterNames[]
        w328 = T5[] []  # All Records
        w329 = T9 refnum  # InverterLUT Dict
        w333 = T11 {"Current VI Reference"=refnum, "Close Panel on Exit?"=FALSE}  # Core
        n154 = Get Date/Time In Seconds() -> (seconds since 1Jan1904=w321:timestamp)
        n155 = local write "LUT File"(path "" ("LUT File")) -> ()
        n156 = Bundle By Name(cluster=w323, "last updated"=w321) -> (w322:T5)
        n157 = Initialize Array(w322, 0 ("dimension size")) -> (w327:T5[])
        n158 = Variant To Data(type=w328, Variant=w327) -> (data=w332:T5[])  [unwired: 1 in, 1 out]
        n159 = call <vilib>:"Create Dynamic CVT Reference.vi"() -> ("dCVT DVR out"=w331:T9)  [unwired: 10 in, 1 out]
        n160 = property on="Inverter List" class="LstBox (strict)"("Item Names"=w325) -> ()  [unwired: 2 in, 2 out]
        n161 = Variant To Data(type=w329, Variant=w331) -> (data=w330:T9)  [unwired: 1 in, 1 out]
        n162 = Bundle("Core"=w333, "CurrInverterRec"=w322, "All Records"=w332, "InverterLUT Dict"=w330) -> (w335:T10)  [unwired: 1 in]
        n163 = call <vilib>:"Add State(s) to Queue__JKI_lib_State_Machine.vi"("State(s) in (\"\")"=w337) -> ("States Out"=w336:string)  [unwired: 14 in]
      }
      frame "Data: Cleanup" {
        n164 = Unbundle By Name(w341) -> ("InverterLUT Dict"=w340:T9, "Core.Current VI Reference"=w344:refnum<vi>)
        n165 = Close Reference(reference=w344, error in (no error)=w343) -> (error out=w342:errorcluster)
        n166 = call <vilib>:"Delete ALL Dynamic CVT Data.vi"("dCVT DVR"=w340) -> ("error out"=w338:errorcluster, "dCVT DVR out"=w339:T9)  [unwired: 9 in]
        n167 = call <vilib>:"Destroy Dynamic CVT Reference.vi"("error in (no error)"=w338, "dCVT DVR"=w339) -> ()  [unwired: 8 in, 2 out]
        n168 = call <vilib>:"Add State(s) to Queue__JKI_lib_State_Machine.vi"("State(s) in (\"\")"=w346) -> ("States Out"=w345:string)  [unwired: 14 in]
      }
      frame "---------- UI ----------" {
        n169 = call <vilib>:"Add State(s) to Queue__JKI_lib_State_Machine.vi"("State(s) in (\"\")"=w350) -> ("States Out"=w349:string)  [unwired: 14 in]
      }
      frame "UI: Warn Dup Records Eliminated" {
        n170 = call <vilib>:"Three Button Dialog.vi"("Window Title (\"\")"="WARNING" ("Window Title (\"\")"), "Center Button Text (\"No\")"="", "message"="Warning: Some records had duplicate Inverter Names.\nInverter Names in the database must be unique.\n\nProceed to update database file with duplicate names removed?\n\nNote: \n<Cancel> terminates editor, and does not modify the database file.\n<Yes> Updates the database file with duplicate Inverter Name records eliminated.") -> ("Which Button?"=w352:T12)  [unwired: 8 in]
        n171 = case shown="\"Left Button\"" w352 {
          tunnel: ["Macro: Exit" "Data: Update Record\nUI: Display Current Record"] -> w351
          frame Default {
          }
          frame "Left Button" {
          }
        }
        n172 = call <vilib>:"Add State(s) to Queue__JKI_lib_State_Machine.vi"("State(s) in Front (\"\")"=w351, "State(s) in (\"\")"=w359) -> ("States Out"=w358:string)  [unwired: 13 in]
      }
      frame "UI: Display Current Record" {
        n173 = Unbundle By Name(w369) -> ("CurrInverterRec"=w368:T5)
        n174 = Unbundle By Name(w368) -> ("name"=w367:string, "last updated"=w362:timestamp, "type"=w380:string, "inverter Info"=w379:T3, "gain range"=w378:T2, "offset range"=w377:T1, "gain actual"=w376:dbl, "offset actual"=w375:dbl, "power level"=w373:dbl, "minimum current"=w374:dbl, "resistance single phase"=w372:dbl, "resistance 3 phase"=w371:dbl, "set flag"=w370:u16)
        n175 = property on="Inverter List" class="LstBox (strict)"() -> ("Item Names"=w366:string[])  [unwired: 2 in, 2 out]
        n176 = local write "inverter Info"(w379) -> ()
        n177 = local write "offset range"(w377) -> ()
        n178 = local write "offset actual"(w375) -> ()
        n179 = local write "minimum current"(w374) -> ()
        n180 = local write "resistance 3 phase"(w371) -> ()
        n181 = Format Date/Time String(seconds (now)=w362) -> (date/time string=w363:string)  [unwired: 2 in]
        n182 = Search 1D Array(1D array=w366, element=w367) -> (index of element=w364:i32)  [unwired: 1 in]
        n183 = local write "Inverter List"(w364) -> ()
        n184 = Increment(x=w364) -> (x+1=w365:i32)
        n185 = local write "name"(w367) -> ()
        n186 = local write "last updated"(w363) -> ()
        n187 = local write "type"(w380) -> ()
        n188 = local write "gain range"(w378) -> ()
        n189 = local write "gain actual"(w376) -> ()
        n190 = local write "power level"(w373) -> ()
        n191 = local write "resistance single phase"(w372) -> ()
        n192 = local write "set flag"(w370) -> ()
        n193 = local write "CurrRec"(w365) -> ()
        n194 = call <vilib>:"Add State(s) to Queue__JKI_lib_State_Machine.vi"("State(s) in (\"\")"=w383) -> ("States Out"=w382:string)  [unwired: 14 in]
      }
      frame "UI: Initialize" {
        n195 = Unbundle By Name(w391) -> ("CurrInverterRec"=w390:T5)
        n196 = Unbundle By Name(w390) -> ("name"=w384:string, "last updated"=w385:timestamp, "type"=w402:string, "inverter Info"=w401:T3, "gain range"=w400:T2, "offset range"=w399:T1, "gain actual"=w398:dbl, "offset actual"=w397:dbl, "power level"=w395:dbl, "minimum current"=w396:dbl, "resistance single phase"=w394:dbl, "resistance 3 phase"=w393:dbl, "set flag"=w392:u16)
        n197 = local write "Total"(0 ("Total")) -> ()
        n198 = local write "CurrRec"(0 ("CurrRec")) -> ()
        n199 = local write "name"(w384) -> ()
        n200 = local write "inverter Info"(w401) -> ()
        n201 = local write "offset range"(w399) -> ()
        n202 = local write "offset actual"(w397) -> ()
        n203 = local write "minimum current"(w396) -> ()
        n204 = local write "resistance 3 phase"(w393) -> ()
        n205 = local write "Inverter List"(-1 ("Inverter List")) -> ()
        n206 = Format Date/Time String(seconds (now)=w385) -> (date/time string=w386:string)  [unwired: 2 in]
        n207 = local write "last updated"(w386) -> ()
        n208 = local write "type"(w402) -> ()
        n209 = local write "gain range"(w400) -> ()
        n210 = local write "gain actual"(w398) -> ()
        n211 = local write "power level"(w395) -> ()
        n212 = local write "resistance single phase"(w394) -> ()
        n213 = local write "set flag"(w392) -> ()
        n214 = call <vilib>:"Add State(s) to Queue__JKI_lib_State_Machine.vi"("State(s) in (\"\")"=w405) -> ("States Out"=w404:string)  [unwired: 14 in]
      }
      frame "UI: OpenFrontPanel" {
        n215 = Unbundle By Name(w415) -> ("Core.Current VI Reference"=w414:refnum<vi>)
        n216 = invoke class="VI" method="FP.Open"(reference=w414, error in=w411, "Activate"=TRUE ("Activate?"), "State"=T8."Standard") -> (reference out=w413:refnum<vi>, error out=w421:errorcluster)  [unwired: 1 in, 3 out]
        n217 = call <userlib>:"MGI Get Executable Version.vi"() -> ("Version"=w407:string)  [unwired: 7 in]
        n218 = Format Into String(format string="Standalone - Inverter LUT UI  [v%s]", w407) -> (resulting string=w406:string)  [unwired: 2 in, 1 out]
        n219 = property class="VI"(reference=w413, error in=w421, "FP.Behavior"=T7."Modal" ("Front Panel Window:Behavior")) -> (reference out=w409:refnum<vi>, error out=w420:errorcluster)
        n220 = property class="VI"(reference=w409, error in=w420, "Front Panel.Title"=w406) -> (error out=w410:errorcluster)  [unwired: 1 out]
        n221 = call <userlib>:"Fit VI window to Largest Dec__ogtk.vi"("error in (no error)"=w410, "border spacing (2 px)"=-2) -> ("error out"=w412:errorcluster)  [unwired: 4 in, 1 out]
        n222 = call <vilib>:"Add State(s) to Queue__JKI_lib_State_Machine.vi"("State(s) in (\"\")"=w423) -> ("States Out"=w422:string)  [unwired: 14 in]
      }
      frame "UI: Cursor Set" {
        # "Argument"
        n223 = case shown="\"Idle\", Default" w424 {
          tunnel: w426 -> [w431 w433]
          tunnel: [w430 w432] -> w425
          frame "Idle", Default {
            n224 = call <vilib>:"Unset Busy.vi"("error in (no error)"=w431) -> ("error out"=w430:errorcluster)  [unwired: 10 in]
          }
          frame "Busy" {
            n225 = call <vilib>:"Set Busy.vi"("error in (no error)"=w433) -> ("error out"=w432:errorcluster)  [unwired: 9 in, 1 out]
          }
        }
        n226 = call <vilib>:"Add State(s) to Queue__JKI_lib_State_Machine.vi"("State(s) in (\"\")"=w429) -> ("States Out"=w428:string)  [unwired: 14 in]
      }
      frame "UI: Front Panel State" {
        # "Use other cases for open/close front panel"
        # "Argument"
        n227 = Unbundle By Name(w436) -> ("Core.Current VI Reference"=w435:refnum<vi>)
        n228 = case shown="\"Open\", Default" w434 {
          tunnel: w438 -> [w444 w457]
          tunnel: [w446 w458] -> w437
          tunnel: w435 -> [w445 w455]
          frame "Open", Default {
            n229 = property class="VI"(reference=w445, error in=w444) -> (reference out=w442:refnum<vi>, error out=w443:errorcluster, "Front Panel.Open"=w441:bool)
            n230 = case shown="False" w441 {
              tunnel: [w449 w452] -> w446
              tunnel: w443 -> [w448 w452]
              tunnel: w442 -> [w447 _]
              frame False {
                n231 = invoke class="VI" method="FP.Open"(reference=w447, error in=w448, "Activate"=TRUE, "State"=T8."Standard") -> (error out=w449:errorcluster)  [unwired: 1 in, 4 out]
              }
              frame True {
              }
            }
          }
          frame "Close" {
            n232 = property class="VI"(reference=w455, error in=w457) -> (reference out=w454:refnum<vi>, error out=w456:errorcluster, "Front Panel.Open"=w453:bool)
            n233 = case shown="True" w453 {
              tunnel: [w459 w462] -> w458
              tunnel: w456 -> [w459 w461]
              tunnel: w454 -> [_ w460]
              frame False {
              }
              frame True {
                n234 = invoke class="VI" method="FP.Close"(reference=w460, error in=w461) -> (error out=w462:errorcluster)  [unwired: 1 in, 2 out]
              }
            }
          }
        }
        n235 = call <vilib>:"Add State(s) to Queue__JKI_lib_State_Machine.vi"("State(s) in (\"\")"=w440) -> ("States Out"=w439:string)  [unwired: 14 in]
      }
      frame "---------- Macro ----------" {
        n236 = call <vilib>:"Add State(s) to Queue__JKI_lib_State_Machine.vi"("State(s) in (\"\")"=w466) -> ("States Out"=w465:string)  [unwired: 14 in]
      }
      frame "Macro: Initialize" {
        n237 = call <vilib>:"Add State(s) to Queue__JKI_lib_State_Machine.vi"("State(s) in Front (\"\")"=w467, "State(s) in (\"\")"=w471) -> ("States Out"=w470:string)  [unwired: 13 in]
      }
      frame "Macro: Exit" {
        n238 = Unbundle By Name(w478) -> ("Core.Close Panel on Exit?"=w477:bool)
        n239 = Select(t="// UI: Front Panel State >> Close", s=w477, f="") -> (s? t:f=w474:string)
        n240 = call <vilib>:"Add State(s) to Queue__JKI_lib_State_Machine.vi"("State(s) in (\"\")"=w474, "State(s) at Back (\"\")"=w472) -> ("States Out"=w473:string)  [unwired: 13 in]
        n241 = call <vilib>:"Add State(s) to Queue__JKI_lib_State_Machine.vi"("State(s) in Front (\"\")"=w473, "State(s) in (\"\")"=w481) -> ("States Out"=w480:string)  [unwired: 13 in]
      }
      frame "---------- Action ----------" {
        n242 = call <vilib>:"Add State(s) to Queue__JKI_lib_State_Machine.vi"("State(s) in (\"\")"=w485) -> ("States Out"=w484:string)  [unwired: 14 in]
      }
      frame "Action: 1" {
        n243 = call <vilib>:"Add State(s) to Queue__JKI_lib_State_Machine.vi"("State(s) in (\"\")"=w489) -> ("States Out"=w488:string)  [unwired: 14 in]
      }
      frame "Action: 2" {
        n244 = call <vilib>:"Add State(s) to Queue__JKI_lib_State_Machine.vi"("State(s) in (\"\")"=w493) -> ("States Out"=w492:string)  [unwired: 14 in]
      }
    }
  }
